vi "LoadPackets.vi"(6 "DefaultFolderName(Data)":string="Data", 7 "DefaultFileExtension(FSDAT)":string="FSDAT") -> (0 "ErrorOut":errorcluster, 3 "Packets":T1[](array[typedef]) {"MeasurementConfig"."Resolution[b]" min=4 max=16 step=1; "MeasurementConfig"."Frequency" min=1 max=10000000 step=1})   [LabVIEW 2016]
doc: "Load packets data from a fall sensor measurement file."
uses:
  Packet.ctl
  Sample.ctl
  Reading.ctl
  MeasurementConfig.ctl
  Measurement/AccelFSRange.ctl
  Measurement/GyroFSRange.ctl
  <vilib>/addons/JSON API/JSON Value/Set from JSON string.vi
  <vilib>/addons/JSON API/JSON Value/JSON Value.lvclass
  <vilib>/addons/JSON API/Get Polymorphic/JSON GetSet.lvlib
panel:
  in  "ErrorIn":errorcluster
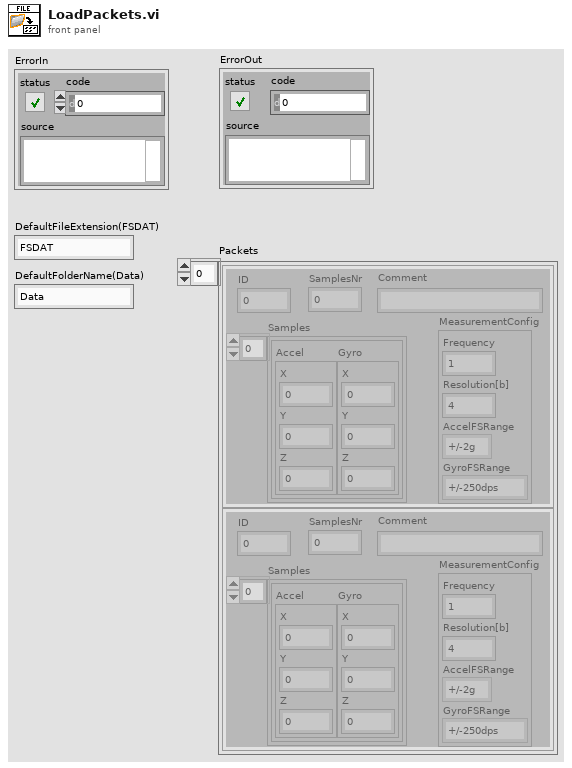
[diagram p1: front panel]
types:
  T1 = typedef "Packet.ctl" = cluster{"ID":u32, "SamplesNr":u32, "Samples":T2[], "MeasurementConfig":T4, "Comment":string}
  T2 = typedef "Sample.ctl" = cluster{"Accel":T3, "Gyro":T3}
  T3 = typedef "Reading.ctl" = cluster{"X":i16, "Y":i16, "Z":i16}
  T4 = typedef "MeasurementConfig.ctl" = cluster{"Frequency":u32, "Resolution[b]":u32, "AccelFSRange":T5, "GyroFSRange":T6}
  T5 = typedef "AccelFSRange.ctl" = enum16{"+/-2g", "+/-4g", "+/-8g", "+/-16g"}
  T6 = typedef "GyroFSRange.ctl" = enum16{"+/-250dps", "+/-500dps", "+/-1000dps", "+/-2000dps"}
  T7 = enum16{"open", "replace", "create", "open or create", "replace or create", "replace or create with confirmation"}
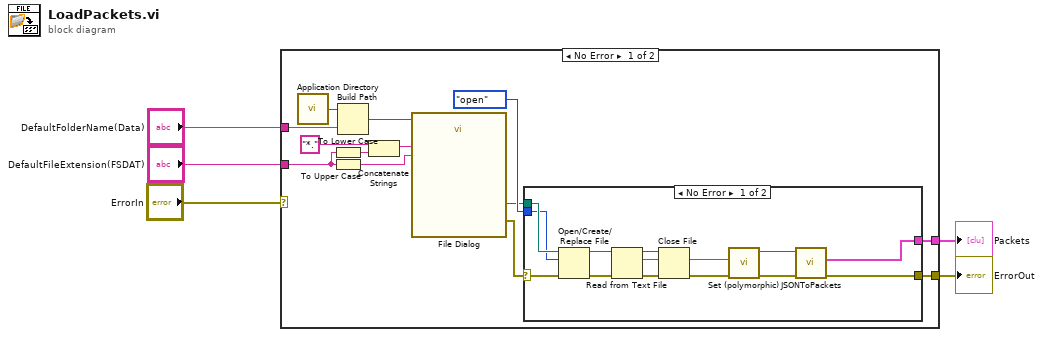
[diagram p0: block diagram]
diagram:
  n1 = case shown="No Error" "ErrorIn" {
    selector: "ErrorIn" -> [_ w33]
    tunnel: "DefaultFolderName(Data)" -> [w18 _]
    tunnel: [w17 w33] -> w4
    tunnel: "DefaultFileExtension(FSDAT)" -> [w16 _]
    tunnel: [w6 _] -> w1
    frame No Error {
      n2 = call <vilib>:"Application Directory.vi"() -> ("Application Directory"=w15:path)
      n3 = To Lower Case(string=w16) -> (all lower case string=w12:string)
      n4 = To Upper Case(1:w16) -> (0:w13:string)
      n5 = Build Path(base path=w15, name or relative path=w18) -> (appended path=w14:path)
      n6 = Concatenate Strings("*." ("string"), w12) -> (w10:string)
      n7 = call "File Dialog"("start path"=w14, "pattern (all files)"=w10, "pattern label"=w13) -> ("selected path"=w8:path, "error out"=w7:errorcluster)  [unwired: 9 in, 2 out]
      n8 = case shown="No Error" w7 {
        selector: w7 -> [w29 w32]
        tunnel: [w19 w32] -> w17
        tunnel: T7."open" ("operation (0:open)") -> [w30 _]
        tunnel: w8 -> [w31 _]
        tunnel: [w20 _] -> w6
        frame No Error {
          n9 = Open/Create/Replace File(file path (use dialog)=w31, error in=w29, operation (0:open)=w30) -> (refnum out=w28:refnum<file>, error out=w27:errorcluster)  [unwired: 3 in, 1 out]
          n10 = Read from Text File(file (use dialog)=w28, error in=w27) -> (refnum out=w26:refnum<file>, text=w24:string, error out=w25:errorcluster)  [unwired: 2 in, 1 out]
          n11 = Close File(refnum=w26, error in=w25) -> (error out=w23:errorcluster)  [unwired: 1 out]
          n12 = call-poly <vilib>:"Set (polymorphic).vi"("error in (no error)"=w23, "JSON stream"=w24) -> ("error out"=w22:errorcluster, "JSON Value out"=w21:refnum<class "JSON Value.lvclass">)  [unwired: 7 in, 1 out]
          n13 = call "JSONToPackets.vi"("ErrorIn"=w22, "JSONIn"=w21) -> ("ErrorOut"=w19:errorcluster, "Packets"=w20:T1[])  [unwired: 7 in, 1 out]
        }
        frame Error {
        }
      }
    }
    frame Error {
    }
  }
  "ErrorOut" <- w4
  "Packets" <- w1
